vi "nodos(SubVI).vi"() -> (3 "Array":string[][](array[string]))   [LabVIEW 2024, in "S7-1200_OPCUA.lvlib"]
uses:
  S7-1200_OPCUA.lvlib
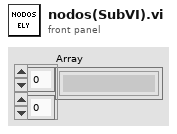
[diagram p1: front panel]
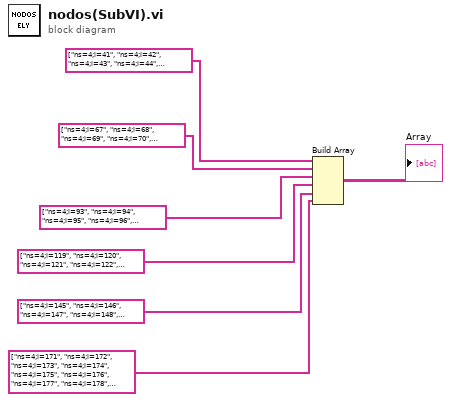
[diagram p0: block diagram]
diagram:
  n1 = Build Array(string[] ["ns=4;i=41", "ns=4;i=42", "ns=4;i=43", "ns=4;i=44", "ns=4;i=45", "ns=4;i=46", "ns=4;i=47", "ns=4;i=48", "ns=4;i=49", "ns=4;i=51", "ns=4;i=52", "ns=4;i=53", "ns=4;i=54", "ns=4;i=55", "ns=4;i=56", "ns=4;i=57", "ns=4;i=58", "ns=4;i=59", "ns=4;i=60", "ns=4;i=61", "ns=4;i=62", "ns=4;i=63"], string[] ["ns=4;i=67", "ns=4;i=68", "ns=4;i=69", "ns=4;i=70", "ns=4;i=71", "ns=4;i=72", "ns=4;i=73", "ns=4;i=74", "ns=4;i=75", "ns=4;i=76", "ns=4;i=77", "ns=4;i=78", "ns=4;i=79", "ns=4;i=80", "ns=4;i=81", "ns=4;i=82", "ns=4;i=83", "ns=4;i=84", "ns=4;i=85", "ns=4;i=86", "ns=4;i=87", "ns=4;i=88", "ns=4;i=89"], string[] ["ns=4;i=93", "ns=4;i=94", "ns=4;i=95", "ns=4;i=96", "ns=4;i=97", "ns=4;i=98", "ns=4;i=99", "ns=4;i=100", "ns=4;i=101", "ns=4;i=102", "ns=4;i=103", "ns=4;i=104", "ns=4;i=105", "ns=4;i=106", "ns=4;i=107", "ns=4;i=108", "ns=4;i=109", "ns=4;i=110", "ns=4;i=111", "ns=4;i=112", "ns=4;i=113", "ns=4;i=114", "ns=4;i=115"], string[] ["ns=4;i=119", "ns=4;i=120", "ns=4;i=121", "ns=4;i=122", "ns=4;i=123", "ns=4;i=124", "ns=4;i=125", "ns=4;i=126", "ns=4;i=127", "ns=4;i=128", "ns=4;i=129", "ns=4;i=130", "ns=4;i=131", "ns=4;i=132", "ns=4;i=133", "ns=4;i=134", "ns=4;i=135", "ns=4;i=136", "ns=4;i=137", "ns=4;i=138", "ns=4;i=139", "ns=4;i=140", "ns=4;i=141"], string[] ["ns=4;i=145", "ns=4;i=146", "ns=4;i=147", "ns=4;i=148", "ns=4;i=149", "ns=4;i=150", "ns=4;i=151", "ns=4;i=152", "ns=4;i=153", "ns=4;i=154", "ns=4;i=155", "ns=4;i=156", "ns=4;i=157", "ns=4;i=158", "ns=4;i=159", "ns=4;i=160", "ns=4;i=161", "ns=4;i=162", "ns=4;i=163", "ns=4;i=164", "ns=4;i=165", "ns=4;i=166", "ns=4;i=167"], string[] ["ns=4;i=171", "ns=4;i=172", "ns=4;i=173", "ns=4;i=174", "ns=4;i=175", "ns=4;i=176", "ns=4;i=177", "ns=4;i=178", "ns=4;i=179", "ns=4;i=180", "ns=4;i=181", "ns=4;i=182", "ns=4;i=183", "ns=4;i=184", "ns=4;i=185", "ns=4;i=186", "ns=4;i=187", "ns=4;i=188", "ns=4;i=189", "ns=4;i=190", "ns=4;i=191", "ns=4;i=192", "ns=4;i=193"]) -> (→"Array":string[][])
